vi "Array of U64_Read Index Set.vi"(9 "Default":cluster{"U64 Array":u64[]}[](array[cluster]), 11 "Indices":i32[](array[numeric])) -> (1 "Values":cluster{"U64 Array":u64[]}[](array[cluster]))   [LabVIEW 2020, in "Current Value Table(Rebuild).lvlib"]
doc: "This VI reads a set of data as defined by the GetIndices function. This VI can provide an order of magnitude increase in performance over a normal index read for sufficiently large data sets."
uses:
  Current Value Table(Rebuild).lvlib
  Type Defs/Memory Commands.ctl
  Array of U64_Memory Block.vi
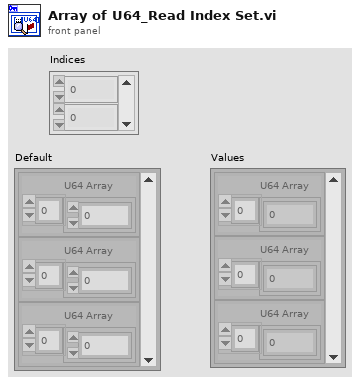
[diagram p1: front panel]
types:
  T1 = typedef "Current Value Table(Rebuild).lvlib/Memory Commands.ctl" = enum16{"Init", "Add Data", "Read", "Read Group", "Read All", "Write", "Write Group", "Get Size"}
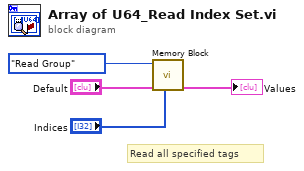
[diagram p0: block diagram]
diagram:
  # "Read all specified tags"
  n1 = call-poly "Memory Block.vi"("Group Indices"="Indices", "Data In"="Default", "Method"=Memory_Commands."Read Group") -> ("Group Data"=→"Values":cluster{"U64 Array":u64[]}[])  [unwired: 6 in, 2 out]
